vi "1.2nad.vi"() -> ()   [LabVIEW 2020]
uses:
  <vilib>/numeric/Random Number (Range) I64.vi
  <vilib>/numeric/sub_Random U32.vi
panel:
  out "Boolean":bool
  out "Numeric":i64
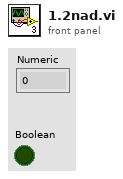
[diagram p1: front panel]
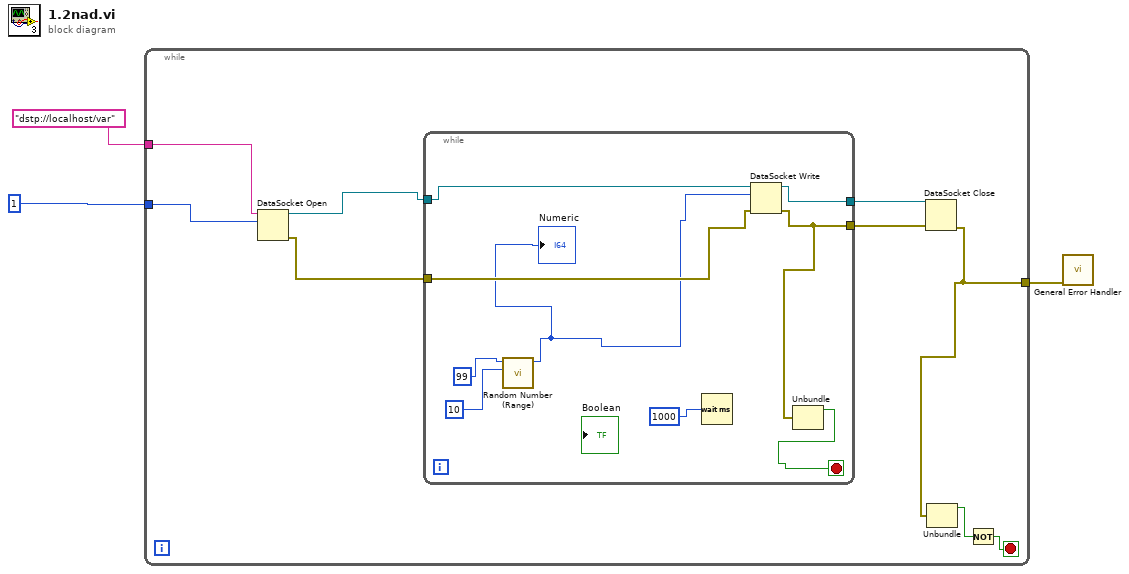
[diagram p0: block diagram]
diagram:
  n1 = while {
    tunnel: 1 -> [w10]
    tunnel: [w5] -> w3
    tunnel: "dstp://localhost/var" -> [w4]
    stop <- w11 stop-if-true
    n2 = DataSocket Open(10:w10, 11:w4) -> (0:w8:errorcluster, 3:w9:refnum<k13>)  [unwired: 2 in]
    n3 = while {
      tunnel: w9 -> [w17]
      tunnel: [w14] -> w7
      tunnel: w8 -> [w16]
      tunnel: [w15] -> w6
      stop <- w18 stop-if-true
      n4 = call-poly <vilib>:"Random Number (Range).vi"("lower bound (-100)"=10, "upper bound (100)"=99) -> ("number"=w13:i64)  [unwired: 9 in]
      "Numeric" <- w13
      n5 = Wait (ms)(milliseconds to wait=1000) -> ()  [unwired: 1 out]
      n6 = DataSocket Write(8:w16, 10:w13, 11:w17) -> (0:w15:errorcluster, 3:w14:refnum<k13>)  [unwired: 1 in, 1 out]
      n7 = Unbundle(w15) -> ("status"=w18:bool)  [unwired: 2 out]
    }
    n8 = DataSocket Close(8:w6, 11:w7) -> (0:w5:errorcluster)  [unwired: 1 in, 1 out]
    n9 = Unbundle(w5) -> ("status"=w12:bool)  [unwired: 2 out]
    n10 = Not(x=w12) -> (.not. x?=w11:bool)
  }
  n11 = call <vilib>:"General Error Handler.vi"("error in (no error)"=w3) -> ()  [unwired: 10 in, 5 out]
